vi "Current time in ics format.vi"(8 "Error In":errorcluster) -> (0 "Error Out":errorcluster, 3 "current time":string)   [LabVIEW 2016]
doc: "This VI returns current time in ics format s"
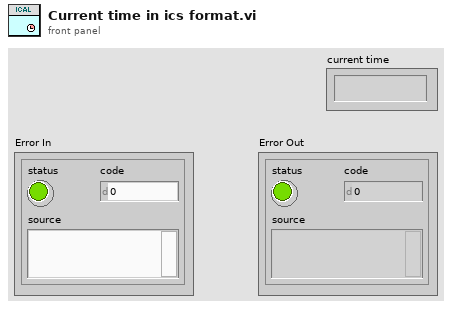
[diagram p1: front panel]
types:
  T1 = typedef "LVDateTimeRec.ctl" = cluster{"fractional second":dbl, "second":i32, "minute":i32, "hour":i32, "day of month":i32, "month":i32, "year":i32, "day of week":i32, "day of year":i32, "DST":i32}
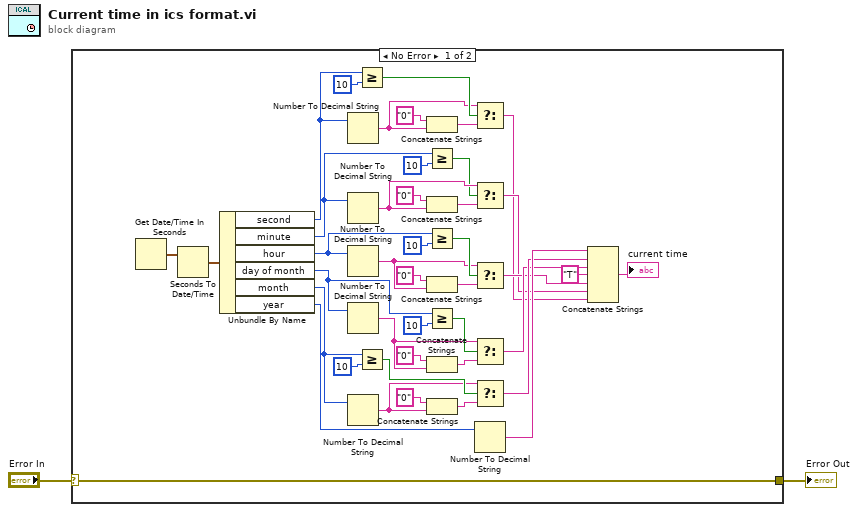
[diagram p0: block diagram]
diagram:
  n1 = case shown="No Error" "Error In" {
    selector: "Error In" -> [w3 w45]
    tunnel: [w3 w45] -> w1
    frame No Error {
      n2 = Get Date/Time In Seconds() -> (seconds since 1Jan1904=w44:timestamp)
      n3 = Seconds To Date/Time(time stamp (now)=w44) -> (date time rec=w43:T1)  [unwired: 1 in]
      n4 = Unbundle By Name(w43) -> ("second"=w30:i32, "minute"=w25:i32, "hour"=w18:i32, "day of month"=w13:i32, "month"=w35:i32, "year"=w42:i32)
      n5 = Number To Decimal String(number=w30) -> (decimal integer string=w31:string)  [unwired: 1 in]
      n6 = Number To Decimal String(number=w25) -> (decimal integer string=w29:string)  [unwired: 1 in]
      n7 = Number To Decimal String(number=w18) -> (decimal integer string=w19:string)  [unwired: 1 in]
      n8 = Number To Decimal String(number=w13) -> (decimal integer string=w37:string)  [unwired: 1 in]
      n9 = Number To Decimal String(number=w35) -> (decimal integer string=w14:string)  [unwired: 1 in]
      n10 = Greater Or Equal?(x=w30, y=10) -> (x >= y?=w34:bool)
      n11 = Greater Or Equal?(x=w35, y=10) -> (x >= y?=w16:bool)
      n12 = Concatenate Strings("0" ("string"), w31) -> (w32:string)
      n13 = Greater Or Equal?(x=w25, y=10) -> (x >= y?=w26:bool)
      n14 = Concatenate Strings("0" ("string"), w29) -> (w28:string)
      n15 = Greater Or Equal?(x=w18, y=10) -> (x >= y?=w22:bool)
      n16 = Concatenate Strings("0" ("string"), w19) -> (w20:string)
      n17 = Greater Or Equal?(x=w13, y=10) -> (x >= y?=w40:bool)
      n18 = Concatenate Strings("0" ("string"), w37) -> (w38:string)
      n19 = Concatenate Strings("0" ("string"), w14) -> (w36:string)
      n20 = Select(t=w31, s=w34, f=w32) -> (s? t:f=w6:string)
      n21 = Select(t=w29, s=w26, f=w28) -> (s? t:f=w7:string)
      n22 = Select(t=w19, s=w22, f=w20) -> (s? t:f=w8:string)
      n23 = Select(t=w37, s=w40, f=w38) -> (s? t:f=w9:string)
      n24 = Select(t=w14, s=w16, f=w36) -> (s? t:f=w10:string)
      n25 = Number To Decimal String(number=w42) -> (decimal integer string=w11:string)  [unwired: 1 in]
      n26 = Concatenate Strings(w11, w10, w9, "T" ("string"), w8, w7, w6) -> (→"current time":string)
    }
    frame Error {
    }
  }
  "Error Out" <- w1
